vi "StopPlay.vi"(8 "error in (no error)":errorcluster, 11 "CameraTestingBL in":refnum<class "CameraTesting.lvclass">) -> (0 "error out":errorcluster, 3 "CameraTestingBL out":refnum<class "CameraTesting.lvclass">)   [LabVIEW 2020, in "CameraTesting.lvlib" / "CameraTesting.lvclass"]
doc: "Send command to camera to stopping the data streaming"
uses:
  CameraTesting.lvclass
  CameraTesting.lvclass/CameraTesting.ctl
  <vilib>/ActorFramework/Message Enqueuer/Message Enqueuer.lvclass/Message Enqueuer.ctl
  <vilib>/ActorFramework/Message Enqueuer/Enqueue.vi
  ICameraTestingUI/ICameraTestingUI Messages/StopPlayRslt Msg/StopPlayRslt Msg.lvclass
  C:/Program Files (x86)/National Instruments/LabVIEW 2020/vi.lib/ActorFramework/Message/Message.lvclass
  <vilib>/ActorFramework/Message Priority Queue/Priority Enqueue.vi
  Camera/ICamera/ICamera/ICamera.lvclass
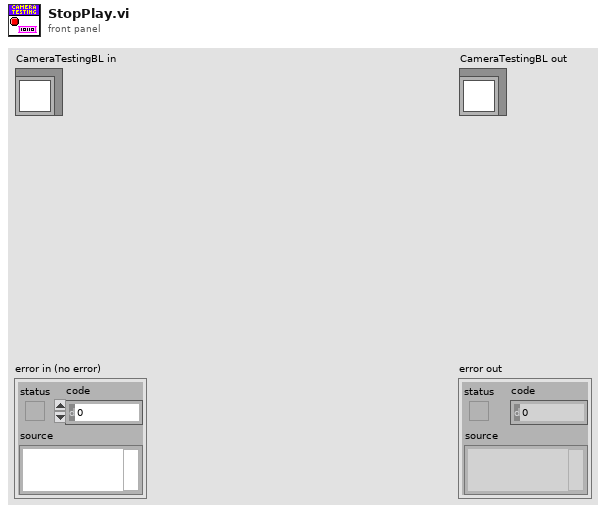
[diagram p1: front panel]
types:
  T1 = typedef "ICameraTesting.lvlib/ICameraTesting.lvclass/StatusUpdated.ctl" = refnum<user-event>
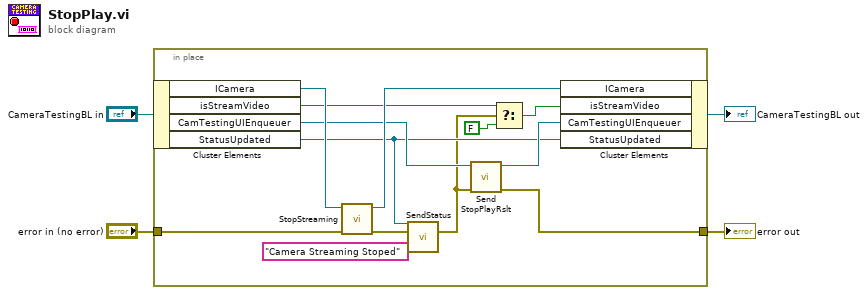
[diagram p0: block diagram]
diagram:
  n1 = in-place {
    in-place-border: [w9] -> w4
    in-place-border: "error in (no error)" -> [w17]
    n2 = in-place-cluster #1("CameraTestingBL in") -> ("ICamera"=w16:refnum<class "ICamera.lvclass">, "isStreamVideo"=w14:bool, "CamTestingUIEnqueuer"=w11:refnum<class "Message Enqueuer.lvclass">, "StatusUpdated"=w6:T1)
    n3 = call-dynamic "StopStreaming.vi"("error in (no error)"=w17, "ICamera in"=w16) -> ("error out"=w7:errorcluster, "ICamera out"=w15:refnum<class "ICamera.lvclass">)  [unwired: 8 in]
    n4 = call "SendStatus.vi"("StatusUsrEvn"=w6, "error in"=w7, "Text"="Camera Streaming Stoped") -> ("error out"=w5:errorcluster)  [unwired: 24 in]
    n5 = call "Send StopPlayRslt.vi"("error in (no error)"=w5, "Message Enqueuer"=w11) -> ("error out"=w9:errorcluster, "Message Enqueuer out"=w10:refnum<class "Message Enqueuer.lvclass">)  [unwired: 8 in]
    n6 = Select(t=w14, s=w5, f=FALSE) -> (s? t:f=w12:bool)
    n7 = in-place-cluster #1("ICamera"=w15, "isStreamVideo"=w12, "CamTestingUIEnqueuer"=w10, "StatusUpdated"=w6) -> (→"CameraTestingBL out":refnum<class "CameraTesting.lvclass">)
  }
  "error out" <- w4
